vi "Datum Size.vi"(1 "datum":T1) -> (0 "size":i32)   [LabVIEW 2020, in "NI_Bytestream.lvlib" / "Bytestream.lvclass"]
uses:
  <vilib>/Array/Bytestream/Bytestream.lvclass
  <vilib>/Array/Bytestream/Datum.ctl
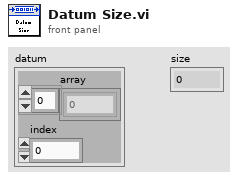
[diagram p1: front panel]
types:
  T1 = typedef "NI_Bytestream.lvlib/Bytestream.lvclass/Datum.ctl" = cluster{"array":u8[], "index":i32}
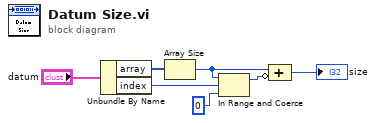
[diagram p0: block diagram]
diagram:
  n1 = Unbundle By Name("datum") -> ("array"=w6:u8[], "index"=w2:i32)
  n2 = Array Size(array=w6) -> (size(s)=w4:i32)
  n3 = In Range and Coerce(upper limit=w4, x=w2, lower limit=0) -> (coerced(x)=w1:i32)  [unwired: 1 out]
  n4 = Compound Arithmetic op=ADD(w4, invert w1) -> (→"size":i32)
